vi "1sec-while.vi"() -> ()   [LabVIEW 2009]
panel:
  out "Numeric 2":i32
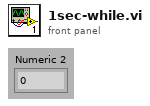
[diagram p1: front panel]
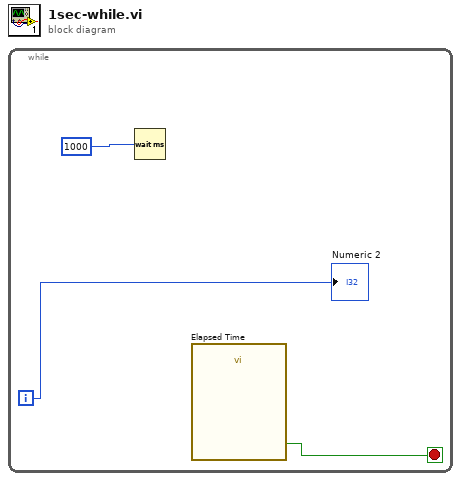
[diagram p0: block diagram]
diagram:
  n1 = while {
    i -> [w1]
    stop <- w3 stop-if-true
    n2 = Wait (ms)(milliseconds to wait=u32 1000) -> ()  [unwired: 1 out]
    n3 = call "Elapsed Time"() -> ("Time has Elapsed"=w3:bool)  [unwired: 12 in, 7 out]
    "Numeric 2" <- w1
  }
